vi "Master, Record Results.vi"(6 "Initialize (F)":bool, 7 "step name":string="Sequence Step General: Name", 8 "error in":errorcluster, 11 "Tbl Refnum":refnum<vi>) -> (0 "error out":errorcluster, 3 "Tbl Refnum dup":refnum<vi>)   [LabVIEW 2010]
panel:
  in  "Test Results":string[][](table) caption="Table 1"
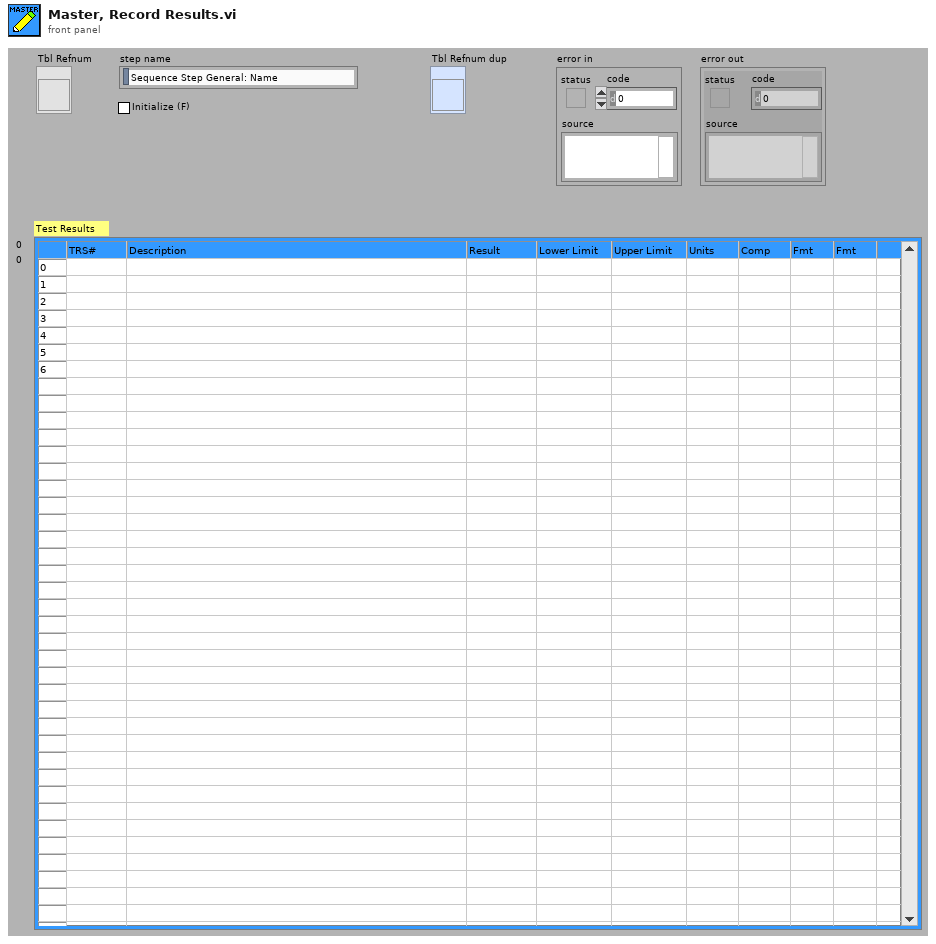
[diagram p1: front panel]
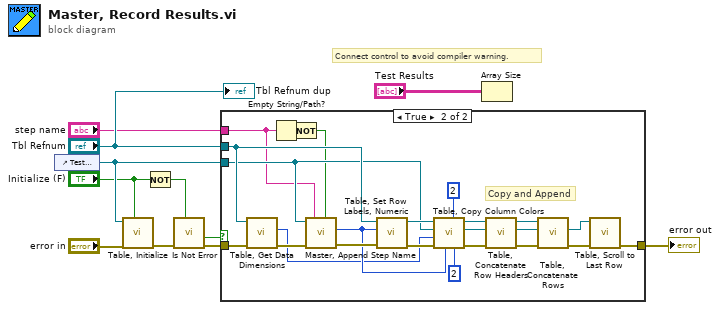
[diagram p0: block diagram]
diagram:
  # "Connect control to avoid compiler warning."
  n1 = control-ref of="Test Results"() -> (w10:refnum<vi>)
  n2 = call "Table, Initialize.vi"("Enable (T)"="Initialize (F)", "error in"="error in", "Tbl Refnum"=w10) -> ("error out"=w7:errorcluster)  [unwired: 7 in, 1 out]
  n3 = Not(x="Initialize (F)") -> (.not. x?=w4:bool)
  n4 = call "Is Not Error.vi"("enable (T)"=w4, "error in"=w7) -> ("error out"=w6:errorcluster, "ready"=w5:bool)  [unwired: 4 in, 1 out]
  n5 = case shown="True" w5 {
    tunnel: w10 -> [_ w17]
    tunnel: "Tbl Refnum" -> [_ w19]
    tunnel: [w12 w34] -> w11
    tunnel: w6 -> [w12 w21]
    tunnel: "step name" -> [_ w16]
    frame False {
    }
    frame True {
      # "Copy and Append"
      n6 = call "Table, Get Data Dimensions.vi"("error in"=w21, "Tbl Refnum"=w19) -> ("error out"=w20:errorcluster, "row_n"=w14:i32)  [unwired: 6 in, 2 out]
      n7 = Empty String/Path?(string/path=w16) -> (empty?=w15:bool)
      n8 = Not(x=w15) -> (.not. x?=w13:bool)
      n9 = call "Master, Append Step Name.vi"("Enable (T)"=w13, "step name"=w16, "error in"=w20, "Tbl Refnum"=w17) -> ("error out"=w29:errorcluster, "row_n (I32)"=w18:i32)  [unwired: 3 in, 1 out]
      n10 = call "Table, Set Row Labels, Numeric.vi"("error in"=w29, "start (0)"=w18, "Tbl Refnum"=w19) -> ("error out"=w28:errorcluster, "Tbl Refnum out"=w26:refnum<vi>)  [unwired: 7 in]
      n11 = call "Table, Copy Column Colors.vi"("dst col (0)"=2 ("src col (0)"), "src col (0)"=2, "dst row (0)"=w18, "error in"=w28, "n rows (1)"=w14, "Tbl Refnum Dst"=w17, "Tbl Refnum Src"=w26) -> ("error out"=w27:errorcluster, "Tbl Refnum Dst out"=w24:refnum<vi>, "Tbl Refnum Src out"=w25:refnum<vi>)  [unwired: 2 in]
      n12 = call "Table, Concatenate Row Headers.vi"("error in"=w27, "Tbl Refnum Dst"=w24, "Tbl Refnum Src"=w25) -> ("error out"=w32:errorcluster, "Tbl Refnum Dst out"=w31:refnum<vi>, "Tbl Refnum Src out"=w30:refnum<vi>)  [unwired: 2 in]
      n13 = call "Table, Concatenate Rows.vi"("error in"=w32, "Tbl Refnum Dst"=w31, "Tbl Refnum Src"=w30) -> ("error out"=w35:errorcluster, "Tbl Refnum Dst out"=w33:refnum<vi>)  [unwired: 2 in, 1 out]
      n14 = call "Table, Scroll to Last Row.vi"("error in"=w35, "Tbl Refnum"=w33) -> ("error out"=w34:errorcluster)  [unwired: 7 in, 2 out]
    }
  }
  "error out" <- w11
  n15 = Array Size(array="Test Results") -> ()  [unwired: 1 out]
  "Tbl Refnum dup" <- "Tbl Refnum"
